vi "In Any Exclude Path.vi"(9 "Exclude Paths":path[](array[path]), 11 "VI Path":path) -> (2 "In Any Exclude Path?":bool)   [LabVIEW 2010]
doc: "<B>Name:</B>\n In Any Exclude Path.vi\n<B>References:</B>\n\n<B>Function Description:</B>\nReturns TRUE if VI Path is in any of the Exclude Paths (or Sub Directories of the Exclude Path), FALSE otherwise.\n\n<B>Inputs:</B>\nVI Path: The path you are querying\nExclude Paths: A list of excluded paths to check\n<B>Outputs:</B>\nIn any excluded path?: Boolean result of search\n<B>Globals:</B>\n\n<B>TestStand Variables:</B>\n\n<B>User Guide:</B>\n\n<B>Control Usage Rules:</B>\n\n<B>VI Interaction:</B>\n\n<B>Occurences:</B>\n\n<B>Devices:</B>\n\n<B>Files:</B>\n\n<B>System Calls:</B>\n\n<B>Keywords:</B>\nexclude, excluded, path\n<B>Initial Developer: Date:</B>\nUjjal Dutt\n\nCurrent Revision: 22\nVSS Version: 3\nCopyright 2002 VI Engineering, Inc."
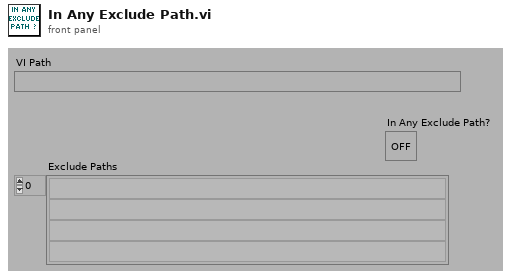
[diagram p1: front panel]
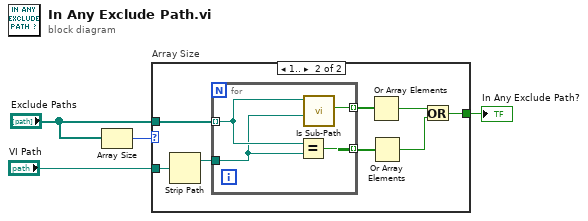
[diagram p0: block diagram]
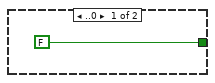
[diagram p2: hidden frame]
diagram:
  n1 = Array Size(array="Exclude Paths") -> (size(s)=w4:i32)
  n2 = case "Array Size" shown="1.." w4 {
    tunnel: "Exclude Paths" -> [_ w11]
    tunnel: "VI Path" -> [_ w10]
    tunnel: [FALSE w6] -> w1
    frame ..0 {
    }
    frame 1.. {
      n3 = Strip Path(path=w10) -> (stripped path=w12:path)  [unwired: 1 out]
      n4 = for {
        tunnel: w11 -> [w16] mode=indexing
        tunnel: [w17] -> w13 mode=indexing
        tunnel: w12 -> [w15]
        tunnel: [w14] -> w9 mode=indexing
        n5 = Equal?(x=w16, y=w15) -> (x = y?=w17:bool)
        n6 = call "Is Sub-Path.vi"("File Path 2"=w15, "File Path"=w16) -> ("File Path 2 a Sub-Path?"=w14:bool)  [unwired: 8 in, 1 out]
      }
      n7 = Or Array Elements(Boolean array=w9) -> (logical OR=w7:bool)
      n8 = Or Array Elements(Boolean array=w13) -> (logical OR=w8:bool)
      n9 = Or(x=w7, y=w8) -> (x .or. y?=w6:bool)
    }
  }
  "In Any Exclude Path?" <- w1
